vi "SMSMagnet.constructor.vi"(0 "name":string, 2 "data in":string, 5 "error in (no error)":errorcluster) -> (14 "i ref out":refnum<vi>, 16 "data out":string, 19 "error out":errorcluster)   [LabVIEW 2014, in "SMSMagnet.lvlib"]
doc: "This is the constructor of a class.\n\nLicense Agreement for this software:\n\nCopyright (C)\nGesellschaft für Schwerionenforschung, GSI\nPlanckstr. 1\n64291 Darmstadt\nGermany\n\nContact: D.Beck@gsi.de \n\nThis program is free software; you can redistribute it and/or modify it under the terms of the \nGNU General Public License as published by the Free Software Foundation; either version 2 of \nthe license, or (at your option) any later version.\n\nThis program is distributed in the hope that it will be useful, but WITHOUT ANY WARRANTY; \nwithout even the implied warranty of MERCHANTABILITY or FITNESS FOR A PARTICULAR PURPOSE. See the GNU General License for more details (http://www.gnu.org).\n\nGesellschaft für Schwerionenforschung, GSI\nPlanckstr. 1, 64291 Darmstadt, Germany\nFor all questions and ideas contact: M.Richter@gsi.de, H.Brand@gsi.de or D.Beck@gsi.de.\nLast update: 16-JUN-2004"
uses:
  SMSMagnet.lvlib
  CSCore/CSApplicationBaseClasses/DeviceBase/DeviceBase.myEventNames.ctl
  CSCore/CSApplicationBaseClasses/DeviceBase/DeviceBase.lvlib
  CSCore/CSSystem/CSSystemLib/CSSystemLib.lvlib
  CSlibraries-extern/DimLVEvent/LVDimInterface/LVDimInterface.lvlib
  CSinstr.lib/SMSMagnetDriver/SMSMagnetDriver.lvlib
  CSCore/BaseProcess/BaseProcess.lvlib
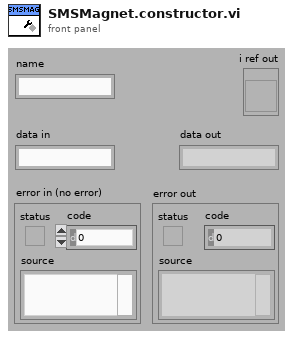
[diagram p1: front panel]
types:
  T1 = enum16{"SetAttribute", "GetAttribute", "CreateAttribute", "DestroyAttribute", "DestroyAllAtributes"}
  T2 = typedef "DeviceBase.lvlib/DeviceBase.myEventNames.ctl" = enum16{"lvmsg://Initialize", "lvmsg://Close", "lvmsg://Configure", "lvmsg://Reset", "lvmsg://IDQuery"}
  T3 = typedef "BaseProcess.lvlib/BaseProcess.i attribute.ctl" = cluster{"EventStatus":string, "EventError":i32, "PresetEvtWatchD":i32, "PresetPdcWatchD":i32, "EventTimeout":i32, "PeriodicInterval":i32, "Interface":string[], "Address":string[], "Special":string[], "PeriodicError":i32, "PeriodicStatus":string, "SuperProc":string, "Descriptors":T4[], "CaseRef":refnum<vi>, "PdcRef":refnum<vi>, "Thread Ref":refnum<vi>, "eventErrorID":i32, "eventStatusID":i32, "periodicErrorID":i32, "periodicStatusID":i32, "pdcCtrID":i32}
  T4 = typedef "BaseProcess.lvlib/BaseProcess.descriptor definition.ctl" = cluster{"selector":string, "descriptor":T5}
  T5 = typedef "BaseProcess.lvlib/BaseProcess.descriptor string definition.ctl" = string
  T6 = typedef "Semaphore RefNum" = refnum<k1>
  T7 = typedef "SMSMagnet.lvlib/SMSMagnet.i attribute.ctl" = cluster{"ActValueID":i32, "NomValueID":i32, "VISA resource name":refnum<visa-resource-name>, "ActValue":dbl, "VISAsem":T6}
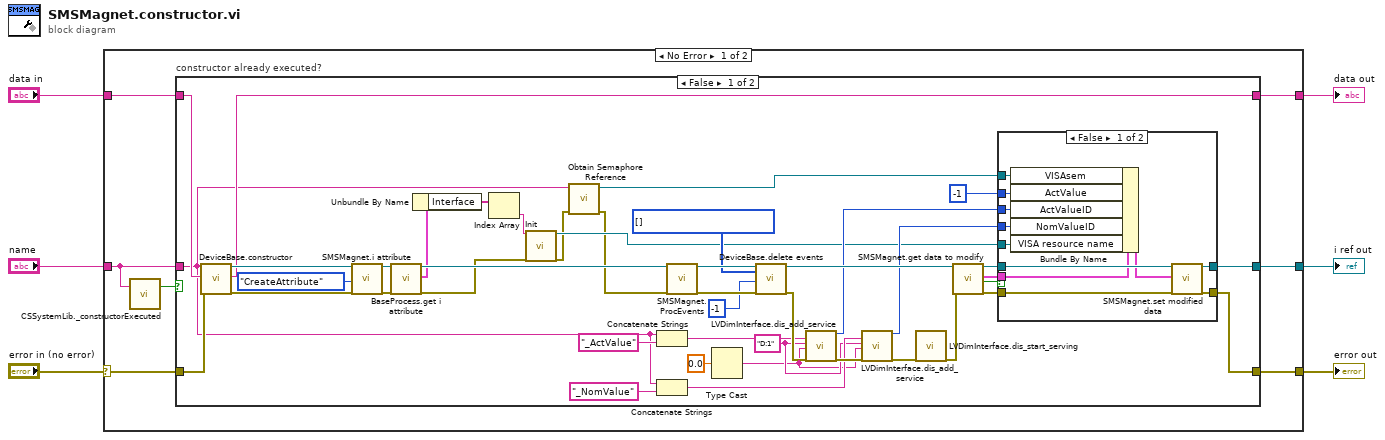
[diagram p0: block diagram]
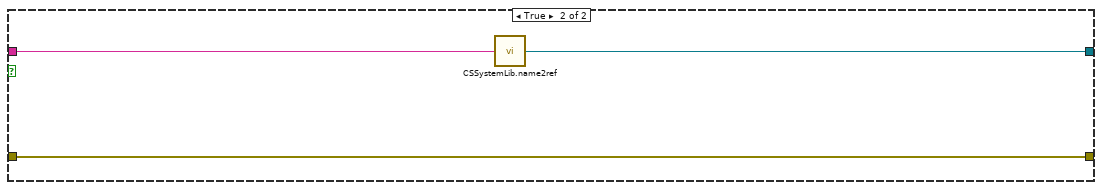
[diagram p3: hidden frame]
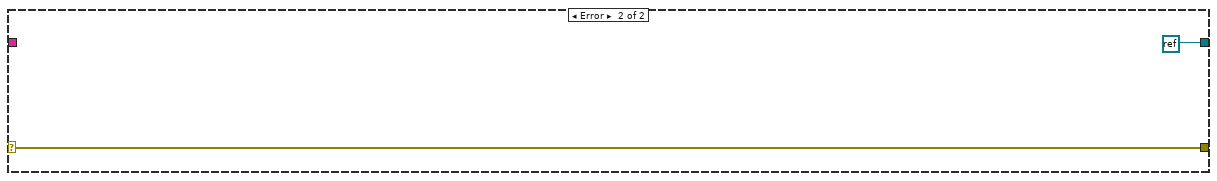
[diagram p4: hidden frame]
diagram:
  n1 = case shown="No Error" "error in (no error)" {
    selector: "error in (no error)" -> [w11 w73]
    tunnel: "name" -> [w10 _]
    tunnel: [w13 refnum<k0> refnum ("Not a Refnum Constant")] -> w5
    tunnel: [w12 w73] -> w4
    tunnel: "data in" -> [w8 _]
    tunnel: [w7 _] -> w1
    frame No Error {
      n2 = call "CSSystemLib._constructorExecuted.vi"("name"=w10) -> ("constructor executed?"=w9:bool)  [unwired: 18 in]
      n3 = case "constructor already executed?" shown="False" w9 {
        tunnel: w10 -> [w15 w72]
        tunnel: [w42 w71] -> w13
        tunnel: [w44 w70] -> w12
        tunnel: w11 -> [w53 w70]
        tunnel: w8 -> [w52 _]
        tunnel: [w47 _] -> w7
        frame False {
          w29 = "D:1" ("typeDescriptor")
          w49 = T2[] [] items=["lvmsg://Initialize", "lvmsg://Close", "lvmsg://Configure", "lvmsg://Reset", "lvmsg://IDQuery"] ("events")
          n4 = call "DeviceBase.constructor.vi"("name"=w15, "data in"=w52, "error in (no error)"=w53) -> ("i ref out"=w56:refnum<vi>, "data out"=w47:string, "error out"=w55:errorcluster)  [unwired: 14 in]
          n5 = call "SMSMagnet.i attribute.vi"("VI Refnum"=w56, "Action"=T1."CreateAttribute", "error in (no error)"=w55) -> ("VI Refnum out"=w25:refnum<vi>, "error out"=w23:errorcluster)  [unwired: 14 in, 1 out]
          n6 = call "BaseProcess.get i attribute.vi"("i ref in"=w25, "error in (no error)"=w23) -> ("i ref out"=w24:refnum<vi>, "i attribute"=w21:T3, "error out"=w22:errorcluster)  [unwired: 15 in]
          n7 = Unbundle By Name(w21) -> ("Interface"=w20:string[])
          n8 = Index Array(array=w20) -> (element=w19:string)  [unwired: 1 in]
          n9 = call "Init.vi"("VISA resource name"=w19, "error in (no error)"=w22) -> ("VISA resource name out"=w26:refnum<visa-resource-name>, "error out"=w17:errorcluster)  [unwired: 16 in]
          n10 = call <vilib>:"Obtain Semaphore Reference.vi"("error in (no error)"=w17, "name (unnamed)"=w15) -> ("error out"=w16:errorcluster, "semaphore"=w14:T6)  [unwired: 3 in, 1 out]
          n11 = Concatenate Strings(w15, "_ActValue" ("string")) -> (w33:string)
          n12 = Concatenate Strings(w15, "_NomValue" ("string")) -> (w32:string)
          n13 = call "SMSMagnet.ProcEvents.vi"("i ref in"=w24, "error in (no error)"=w16) -> ("i ref out"=w51:refnum<vi>, "error out"=w50:errorcluster)  [unwired: 16 in]
          n14 = Type Cast(x=0.0) -> (*(type *) &x=w27:string)  [unwired: 1 in]
          n15 = call "DeviceBase.delete events.vi"("i ref in"=w51, "events"=w49, "ms timeout (10000)"=-1, "error in (no error)"=w50) -> ("i ref out"=w46:refnum<vi>, "error out"=w39:errorcluster)  [unwired: 13 in, 1 out]
          n16 = call "LVDimInterface.dis_add_service.vi"("serviceName"=w33, "typeDescriptor"=w29, "data"=w27, "error in (no error)"=w39) -> ("my_serviceID"=w34:i32, "error out"=w38:errorcluster)  [unwired: 14 in]
          n17 = call "LVDimInterface.dis_add_service.vi"("serviceName"=w32, "typeDescriptor"=w29, "data"=w27, "error in (no error)"=w38) -> ("my_serviceID"=w35:i32, "error out"=w37:errorcluster)  [unwired: 14 in]
          n18 = call "LVDimInterface.dis_start_serving.vi"("error in (no error)"=w37) -> ("error out"=w36:errorcluster)  [unwired: 17 in, 1 out]
          n19 = call "SMSMagnet.get data to modify.vi"("i ref in"=w46, "error in (no error)"=w36) -> ("i ref out"=w43:refnum<vi>, "i attribute"=w40:T7, "timed out"=w41:bool, "error out"=w45:errorcluster)  [unwired: 14 in]
          n20 = case shown="False" w41 {
            tunnel: w45 -> [w67 w68]
            tunnel: [w66 w68] -> w44
            tunnel: w43 -> [w65 w69]
            tunnel: [w64 w69] -> w42
            tunnel: w40 -> [w63 _]
            tunnel: w35 -> [w61 _]
            tunnel: w34 -> [w60 _]
            tunnel: w26 -> [w59 _]
            tunnel: -1 -> [w58 _]
            tunnel: w14 -> [w57 _]
            frame False {
              n21 = Bundle By Name(cluster=w63, "VISAsem"=w57, "ActValue"=w58, "ActValueID"=w60, "NomValueID"=w61, "VISA resource name"=w59) -> (w62:T7)
              n22 = call "SMSMagnet.set modified data.vi"("i ref in"=w65, "i attribute"=w62, "error in (no error)"=w67) -> ("i ref out"=w64:refnum<vi>, "error out"=w66:errorcluster)  [unwired: 15 in]
            }
            frame True {
            }
          }
        }
        frame True {
          n23 = call "CSSystemLib.name2ref.vi"("name"=w72) -> ("obj refnum"=w71:refnum<vi>)
        }
      }
    }
    frame Error {
    }
  }
  "i ref out" <- w5
  "error out" <- w4
  "data out" <- w1
